vi "CAM String Array.vi"() -> (3 "CAM string array":i8[][](array[numeric]))   [LabVIEW 2023, in "Vision.lvlib"]
uses:
  Vision/Vision.lvlib
  bin/Vision.dll
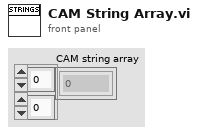
[diagram p1: front panel]
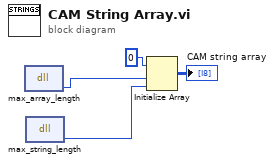
[diagram p0: block diagram]
diagram:
  n1 = dll-call lib="C:/Users/cfangmeier3/Desktop/nebraska-silicon-lab/pixel-gantry-control/Gantry/Shared Components/bin/Vision.dll" fn="max_array_length"() -> ("return type"=w3:i32)  [unwired: 3 in, 2 out]
  n2 = dll-call lib="C:/Users/cfangmeier3/Desktop/nebraska-silicon-lab/pixel-gantry-control/Gantry/Shared Components/bin/Vision.dll" fn="max_string_length"() -> ("return type"=w2:i32)  [unwired: 3 in, 2 out]
  n3 = Initialize Array(i8 0 ("element"), w3, w2) -> (→"CAM string array":i8[][])
